vi "picktime.vi"(7 "first":i32 caption="第一", 8 "wdnames":string[](array[string])=["日", "一", "二", "三", "四", "五", "六"] caption="星期名称", 9 "fmtstr":string="%<%X\n%x>T" caption="格式字符串", 10 "secin":timestamp caption="秒输入", 11 "mnames":string[](array[string])=["一月", "二月", "三月", "四月", "五月", "六月", "七月", "八月", "九月", "十月", "十一月", "十二月"] caption="月份名称") -> (1 "ok":bool caption="确定", 2 "secout":timestamp caption="秒输出" format="%<%Z>T")   [LabVIEW 2016]
uses:
  <vilib>/Utility/miscctls.llb/LVPointTypeDef.ctl
panel:
  in  "help":bool caption="取消"
  out "DaylightSavingState":string caption="夏令时状态"
  out "date time rec":T1 caption="日期时间记录"
  in  "Time Display":timestamp caption="时间显示" format="%<%X>T"
  in  "now":bool caption="现在"
  in  "cancel":bool caption="取消"
  in  "ok":bool caption="确定"
  in  "Year":i32=1905 caption="年" min=1600 max=3000
  in  "Month":i32(ring) caption="月" items=["一月", "二月", "三月", "四月", "五月", "六月", "七月", "八月", "九月", "十月", "十一月", "十二月"]
  in  "Date":i32(listbox) caption="日期"
  # "（0表示星期天，1表示星期一，等）"
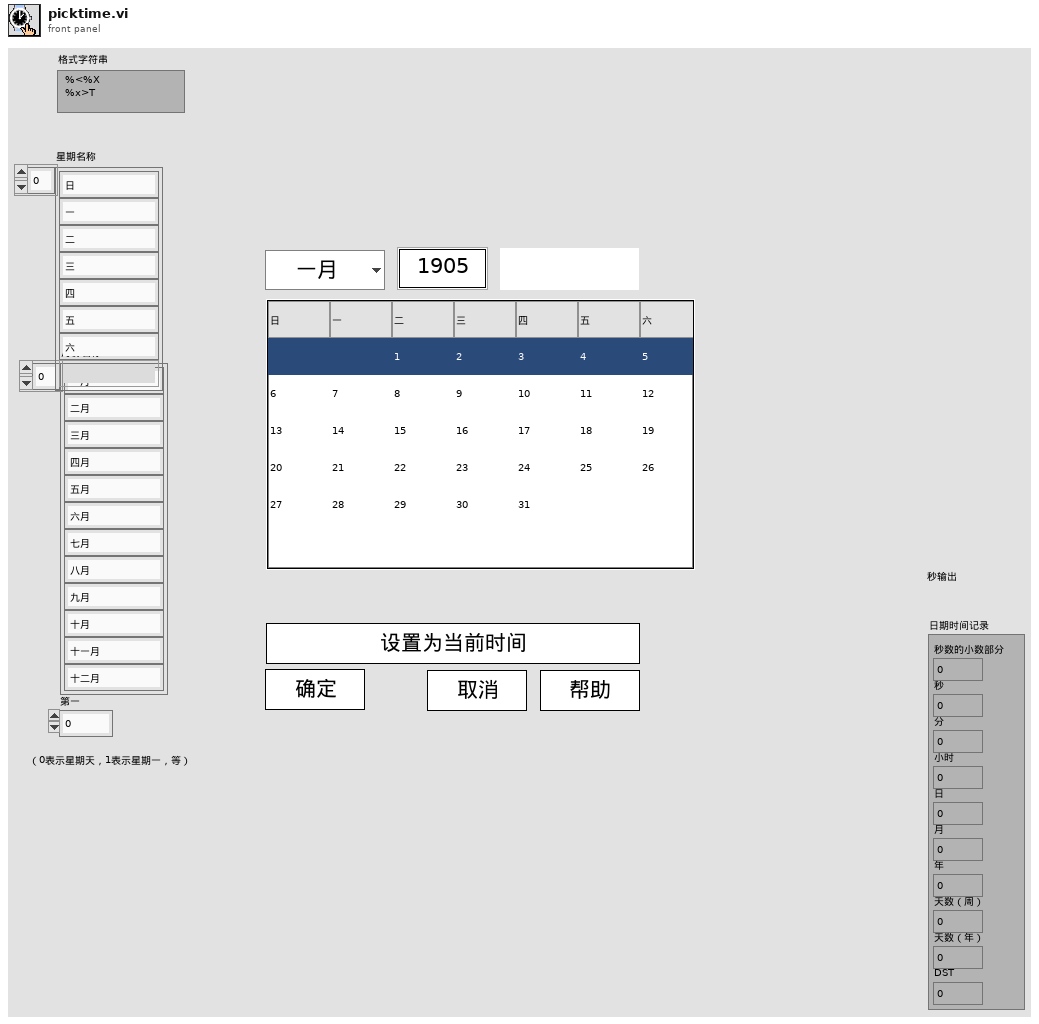
[diagram p1: front panel]
types:
  T1 = cluster{"fractional second":dbl, "second":i32, "minute":i32, "hour":i32, "day of month":i32, "month":i32, "year":i32, "day of week":i32, "day of year":i32, "DST":i32}
  T2 = typedef "LVPointTypeDef.ctl" = cluster{"Horizontal":i16, "Vertical":i16}
  T3 = typedef "LVDateTimeRec.ctl" = cluster{"fractional second":dbl, "second":i32, "minute":i32, "hour":i32, "day of month":i32, "month":i32, "year":i32, "day of week":i32, "day of year":i32, "DST":i32}
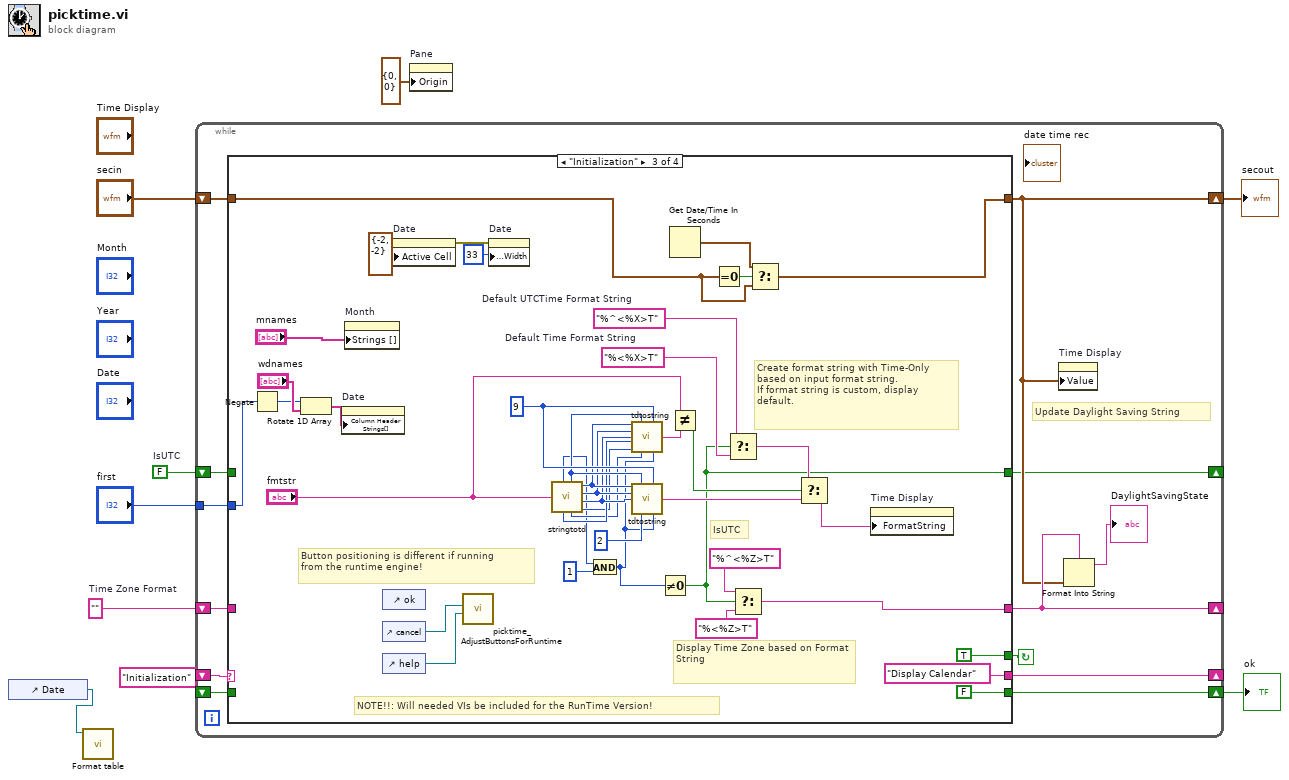
[diagram p0: block diagram]
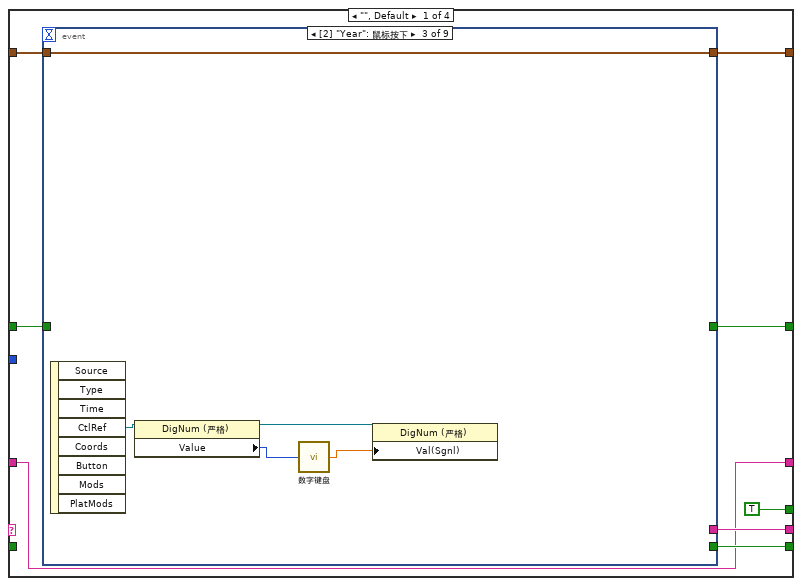
[diagram p2: hidden frame]
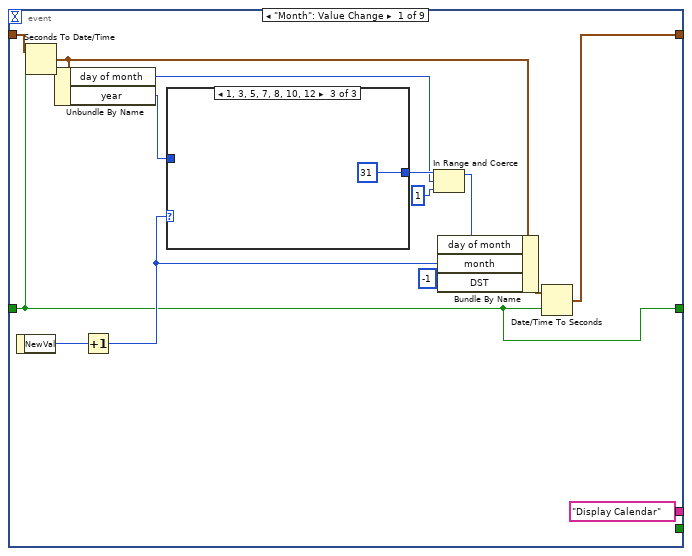
[diagram p3: hidden frame]
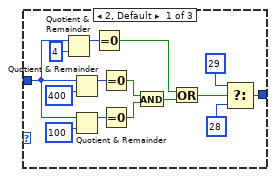
[diagram p4: hidden frame]
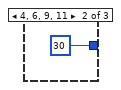
[diagram p5: hidden frame]
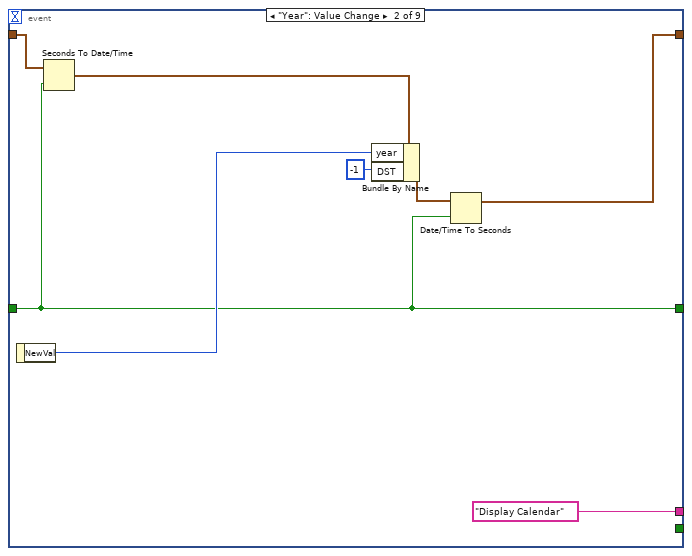
[diagram p6: hidden frame]
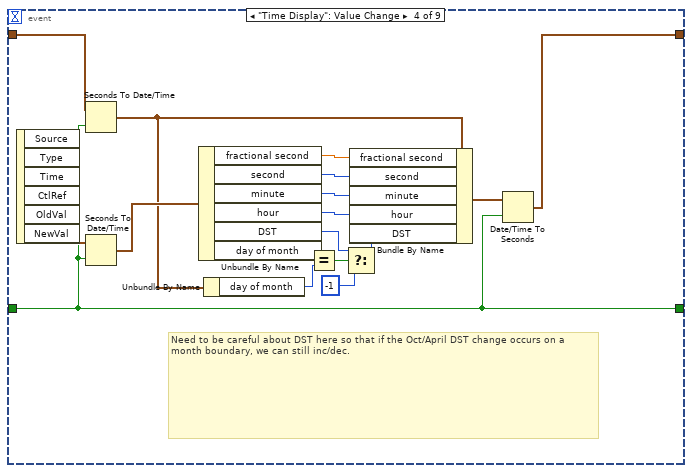
[diagram p7: hidden frame]
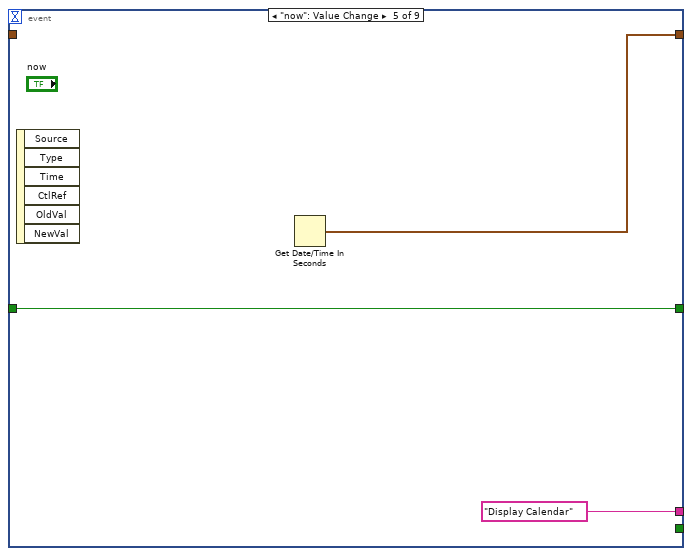
[diagram p8: hidden frame]
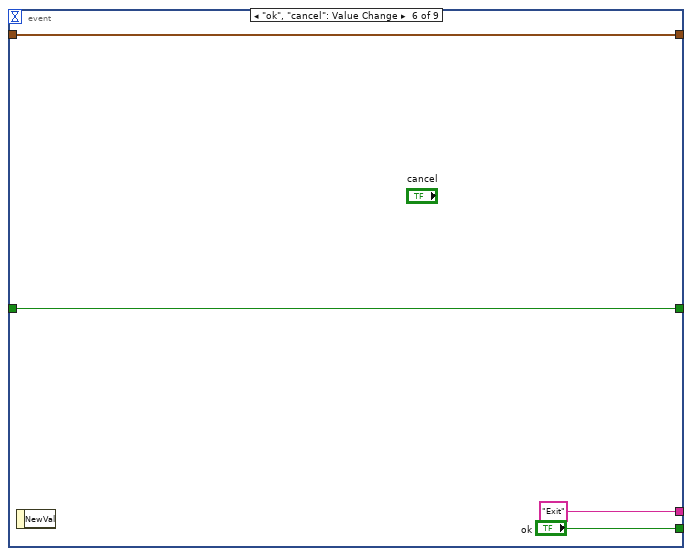
[diagram p9: hidden frame]
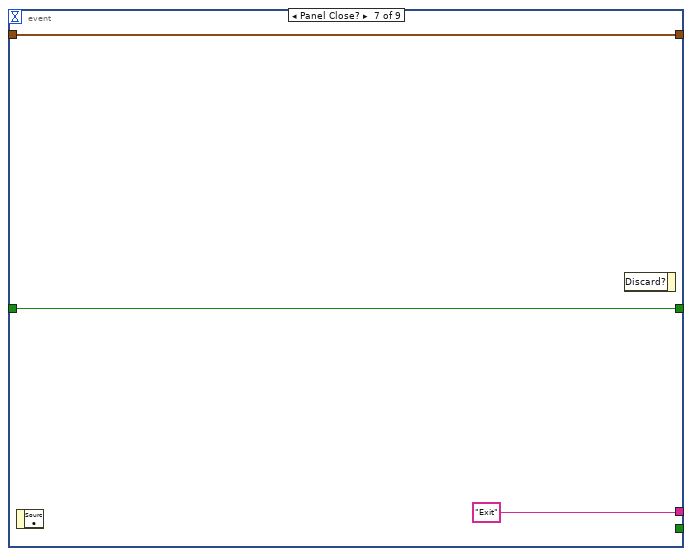
[diagram p10: hidden frame]
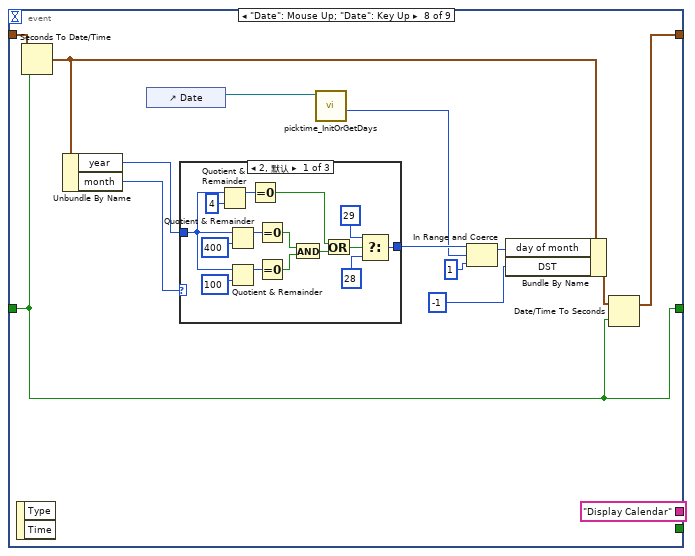
[diagram p11: hidden frame]
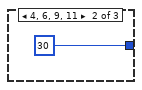
[diagram p12: hidden frame]
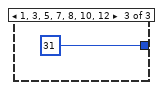
[diagram p13: hidden frame]
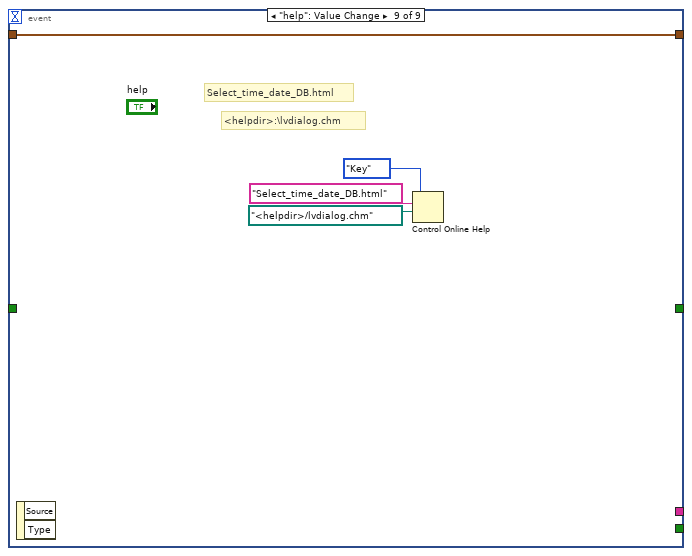
[diagram p14: hidden frame]
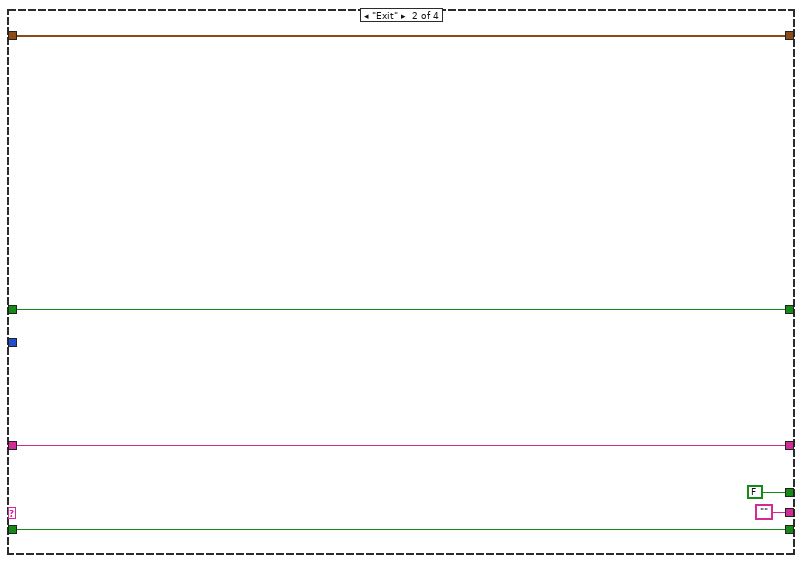
[diagram p15: hidden frame]
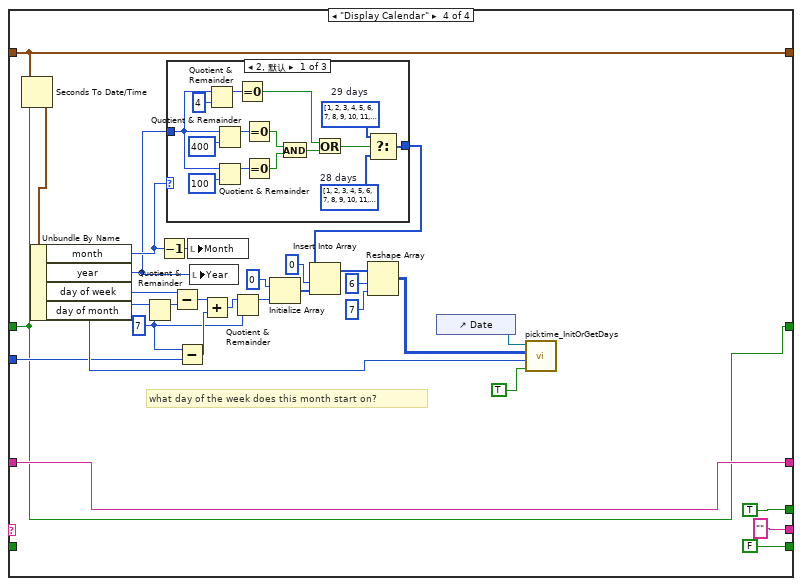
[diagram p16: hidden frame]
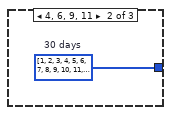
[diagram p17: hidden frame]
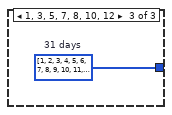
[diagram p18: hidden frame]
diagram:
  w3 = FALSE  # IsUTC
  w5 = ""  # Time Zone Format
  n1 = control-ref of="Date"() -> (w2:refnum<vi>)
  n2 = call "Format table.vi"("Table输入"=w2) -> ()  [unwired: 11 in]
  n3 = while {
    shift-right: [w21] -> _
    shift-left: "Initialization" -> [w22]
    shift-right: [w13] -> w6
    shift-left: "secin" -> [w20]
    shift-right: [w18] -> w8
    shift-left: _ -> [w17]
    shift-right: [w14] -> _
    shift-left: w5 -> [w16]
    tunnel: "first" -> [w12]
    shift-right: [w10] -> _
    shift-left: w3 -> [w11]
    stop <- w19 continue-if-true
    # "Update Daylight Saving String"
    n4 = case shown="\"Initialization\"" w22 {
      tunnel: [w27 "" "Display Calendar" ""] -> w21
      tunnel: [TRUE FALSE TRUE TRUE] -> w19
      tunnel: w20 -> [w28 w139 w174 w194]
      tunnel: [w29 w139 w173 w194] -> w13
      tunnel: [w26 w140 FALSE ("ok") FALSE ("ok")] -> w18
      tunnel: w17 -> [_ w140 _ _]
      tunnel: [w25 w138 w153 w193] -> w14
      tunnel: w16 -> [w25 w138 _ w193]
      tunnel: w12 -> [_ _ w149 w189]
      tunnel: w11 -> [w24 w137 _ w186]
      tunnel: [w23 w137 w147 w186] -> w10
      frame "", Default {
        n5 = event shown="[2] \"Year\": 鼠标按下" {
          selector: _ -> [_ _ _ _ _ _ _ _ _]
          dyn-events: _ -> [_ _ _ _ _ _ _ _ _]
          timeout: _ -> [_ _ _ _ _ _ _ _ _]
          tunnel: w28 -> [w34 w65 w74 w90 _ w96 w100 w107 w136]
          tunnel: [w33 w63 w74 w88 w93 w96 w100 w105 w136] -> w29
          tunnel: ["Display Calendar" "Display Calendar" _ _ "Display Calendar" "Exit" "Exit" "Display Calendar" _] -> w27
          tunnel: [_ _ _ _ _ "ok" _ _ _] -> w26
          tunnel: w24 -> [w31 w62 _ w75 w92 w95 w99 w104 _]
          tunnel: [w31 w62 _ w75 w92 w95 w99 w104 _] -> w23
          event "Month": Value Change {
            n6 = event-data() -> ("NewVal"=w44:i32)  [unwired: 1 out]
            n7 = Seconds To Date/Time(time stamp (now)=w34, to UTC (F)=w31) -> (date time rec=w32:T3)
            n8 = Unbundle By Name(w32) -> ("day of month"=w38:i32, "year"=w39:i32)
            n9 = Increment(x=w44) -> (x+1=w42:i32)
            n10 = case shown="1, 3, 5, 7, 8, 10, 12" w42 {
              tunnel: [w57 30 31] -> w41
              tunnel: w39 -> [w52 _ _]
              frame 2, Default {
                n11 = Quotient & Remainder(x=w52, y=4) -> (x-y*floor(x/y)=w56:i32)  [unwired: 1 out]
                n12 = Quotient & Remainder(x=w52, y=400) -> (x-y*floor(x/y)=w51:i32)  [unwired: 1 out]
                n13 = Quotient & Remainder(x=w52, y=100) -> (x-y*floor(x/y)=w50:i32)  [unwired: 1 out]
                n14 = Equal To 0?(x=w56) -> (x = 0?=w55:bool)
                n15 = Equal To 0?(x=w51) -> (x = 0?=w48:bool)
                n16 = Equal To 0?(x=w50) -> (x = 0?=w49:bool)
                n17 = And(x=w48, y=w49) -> (x .and. y?=w47:bool)
                n18 = Or(x=w55, y=w47) -> (x .or. y?=w54:bool)
                n19 = Select(t=29, s=w54, f=28) -> (s? t:f=w57:i32)
              }
              frame 4, 6, 9, 11 {
              }
              frame 1, 3, 5, 7, 8, 10, 12 {
              }
            }
            n20 = In Range and Coerce(upper limit=w41, x=w38, lower limit=1) -> (coerced(x)=w37:i32)  [unwired: 1 out]
            n21 = Bundle By Name(cluster=w32, "day of month"=w37, "month"=w42, "DST"=-1) -> (w36:T3)
            n22 = Date/Time To Seconds(1:w31, 2:w36) -> (0:w33:timestamp)
          }
          event "Year": Value Change {
            n23 = event-data() -> ("NewVal"=w69:i32)  [unwired: 1 out]
            n24 = Seconds To Date/Time(time stamp (now)=w65, to UTC (F)=w62) -> (date time rec=w64:T3)
            n25 = Bundle By Name(cluster=w64, "year"=w69, "DST"=-1) -> (w67:T3)
            n26 = Date/Time To Seconds(1:w62, 2:w67) -> (0:w63:timestamp)
          }
          event "Year": Mouse Down {
            n27 = event-data() -> ("CtlRef"=w73:refnum<vi>)  [unwired: 8 out]
            n28 = property class="DigNum (严格)"(reference=w73) -> (reference out=w71:refnum<vi>, "Value"=w72:i32)  [unwired: 1 in, 1 out]
            n29 = call "数字键盘.vi"("OldNumber"=w72) -> ("NewNumber"=w70:sgl)
            n30 = property class="DigNum (严格)"(reference=w71, "Val(Sgnl)"=w70) -> ()  [unwired: 1 in, 2 out]
          }
          event "Time Display": Value Change {
            # "Need to be careful about DST here so that if the Oct/April DST change occurs on a month boundary, we can still inc/dec."
            n31 = event-data() -> ("NewVal"=w91:timestamp)  [unwired: 6 out]
            n32 = Seconds To Date/Time(time stamp (now)=w90, to UTC (F)=w75) -> (date time rec=w78:T3)
            n33 = Seconds To Date/Time(time stamp (now)=w91, to UTC (F)=w75) -> (date time rec=w87:T3)
            n34 = Unbundle By Name(w87) -> ("fractional second"=w83:dbl, "second"=w84:i32, "minute"=w85:i32, "hour"=w86:i32, "DST"=w80:i32, "day of month"=w76:i32)
            n35 = Unbundle By Name(w78) -> ("day of month"=w77:i32)
            n36 = Equal?(x=w76, y=w77) -> (x = y?=w82:bool)
            n37 = Select(t=w80, s=w82, f=-1) -> (s? t:f=w79:i32)
            n38 = Bundle By Name(cluster=w78, "fractional second"=w83, "second"=w84, "minute"=w85, "hour"=w86, "DST"=w79) -> (w89:T3)
            n39 = Date/Time To Seconds(1:w75, 2:w89) -> (0:w88:timestamp)
          }
          event "now": Value Change {
            n40 = event-data() -> ()  [unwired: 7 out]
            n41 = Get Date/Time In Seconds() -> (seconds since 1Jan1904=w93:timestamp)
          }
          event "ok", "cancel": Value Change {
            n42 = event-data() -> ()  [unwired: 2 out]
          }
          event Panel Close? {
            n43 = event-data() -> ()  [unwired: 2 out]
            n44 = event-data() -> ()  [unwired: 1 in, 2 out]
          }
          event "Date": Mouse Up; "Date": Key Up {
            n45 = event-data() -> ()  [unwired: 3 out]
            n46 = Seconds To Date/Time(time stamp (now)=w107, to UTC (F)=w104) -> (date time rec=w106:T3)
            n47 = Unbundle By Name(w106) -> ("year"=w113:i32, "month"=w112:i32)
            n48 = control-ref of="Date"() -> (w102:refnum<vi>)
            n49 = case shown="2, 默认" w112 {
              tunnel: [w128 30 31] -> w115
              tunnel: w113 -> [w123 _ _]
              frame 2, Default {
                n50 = Quotient & Remainder(x=w123, y=4) -> (x-y*floor(x/y)=w127:i32)  [unwired: 1 out]
                n51 = Quotient & Remainder(x=w123, y=400) -> (x-y*floor(x/y)=w122:i32)  [unwired: 1 out]
                n52 = Quotient & Remainder(x=w123, y=100) -> (x-y*floor(x/y)=w121:i32)  [unwired: 1 out]
                n53 = Equal To 0?(x=w127) -> (x = 0?=w126:bool)
                n54 = Equal To 0?(x=w122) -> (x = 0?=w119:bool)
                n55 = Equal To 0?(x=w121) -> (x = 0?=w120:bool)
                n56 = And(x=w119, y=w120) -> (x .and. y?=w118:bool)
                n57 = Or(x=w126, y=w118) -> (x .or. y?=w125:bool)
                n58 = Select(t=29, s=w125, f=28) -> (s? t:f=w128:i32)
              }
              frame 4, 6, 9, 11 {
              }
              frame 1, 3, 5, 7, 8, 10, 12 {
              }
            }
            n59 = call <resource>:"picktime_InitOrGetDays.vi"("reference"=w102) -> ("day of month(out)"=w103:i32)  [unwired: 3 in, 7 out]
            n60 = In Range and Coerce(upper limit=w115, x=w103, lower limit=1) -> (coerced(x)=w111:i32)  [unwired: 1 out]
            n61 = Bundle By Name(cluster=w106, "day of month"=w111, "DST"=-1) -> (w109:T3)
            n62 = Date/Time To Seconds(1:w104, 2:w109) -> (0:w105:timestamp)
          }
          event "help": Value Change {
            # "<helpdir>:\\lvdialog.chm"
            # "Select_time_date_DB.html"
            n63 = event-data() -> ()  [unwired: 3 out]
            n64 = Control Online Help(2:path "<helpdir>/lvdialog.chm" ("Path to the help file"), 3:"Select_time_date_DB.html" ("String to search for"), 4:enum16{"Contents", "Key", "Close"}."Key" ("Operation")) -> ()  [unwired: 1 in, 1 out]
          }
        }
      }
      frame "Exit" {
      }
      frame "Initialization" {
        w156 = "%^<%X>T"  # Default UTCTime Format String
        w155 = "%<%X>T"  # Default Time Format String
        w169 = 9 ("Type (9 = Absolute)")
        # "Button positioning is different if running\nfrom the runtime engine!"
        # "IsUTC"
        # "Display Time Zone based on Format String"
        # "NOTE!!: Will needed VIs be included for the RunTime Version!"
        # "Create format string with Time-Only based on input format string.\nIf format string is custom, display default."
        n65 = Negate(x=w149) -> (-x=w148:i32)
        n66 = Rotate 1D Array(1:"wdnames", 2:w148) -> (0:w151:string[])
        n67 = property on="Date" class="MCListbox (严格)"("Column Header Strings[]"=w151) -> ()  [unwired: 2 in, 2 out]
        n68 = property on="Month" class="Ring (严格)"("Strings []"="mnames") -> ()  [unwired: 2 in, 2 out]
        n69 = control-ref of="ok"() -> ()  [unwired: 1 out]
        n70 = control-ref of="cancel"() -> (w144:refnum<vi>)
        n71 = control-ref of="help"() -> (w143:refnum<vi>)
        n72 = property on="Date" class="MCListbox (严格)"("Active Cell"=cluster{i32, i32} {-2, -2}) -> (error out=w181:errorcluster)  [unwired: 2 in, 1 out]
        n73 = call <resource>:"picktime_AdjustButtonsForRuntime.vi"("help button ref"=w143, "cancel button ref"=w144) -> ()  [unwired: 1 in, 9 out]
        n74 = property on="Date" class="MCListbox (严格)"(error in=w181, "Cell Size:Width"=u32 33) -> ()  [unwired: 1 in, 2 out]
        n75 = call <resource>:"stringtotd.vi"("Time & Date Format String"="fmtstr") -> ("UTC"=w145:i16, "MDY"=w164:i16, "Time Format"=w168:i16, "AM/PM"=w167:i16, "included seconds"=w166:i16, "Date Format"=w162:i16, "seconds precision"=w165:i16, "Year Format"=w163:i16)  [unwired: 2 out]
        n76 = And(x=w145, y=i16 1) -> (x .and. y?=w146:i16)
        n77 = call <resource>:"tdtostring.vi"("AM/PM"=w167, "Time Format"=w168, "Type (10 = Absolute)"=w169, "included seconds"=w166, "seconds precision"=w165, "m-d-y sequence"=w164, "year format"=w163, "Date Format"=w162, "UTC"=w146) -> ("Format String"=w160:string)  [unwired: 2 in, 4 out]
        n78 = call <resource>:"tdtostring.vi"("AM/PM"=w167, "Time Format"=w168, "Type (10 = Absolute)"=w169, "included seconds"=w166, "seconds precision"=w165, "Date Format"=i16 2, "UTC"=w146) -> ("Format String"=w158:string)  [unwired: 4 in, 4 out]
        n79 = Not Equal To 0?(x=w146) -> (x != 0?=w147:bool)
        n80 = Get Date/Time In Seconds() -> (seconds since 1Jan1904=w176:timestamp)
        n81 = Not Equal?(x="fmtstr", y=w160) -> (x != y?=w159:bool)
        n82 = Equal To 0?(x=w174) -> (x = 0?=w177:bool)
        n83 = Select(t=w156, s=w147, f=w155) -> (s? t:f=w154:string)
        n84 = Select(t="%^<%Z>T", s=w147, f="%<%Z>T") -> (s? t:f=w153:string)
        n85 = Select(t=w176, s=w177, f=w174) -> (s? t:f=w173:timestamp)
        n86 = Select(t=w154, s=w159, f=w158) -> (s? t:f=w157:string)
        n87 = property on="Time Display" class="AbsTime (严格)"("FormatString"=w157) -> ()  [unwired: 2 in, 2 out]
      }
      frame "Display Calendar" {
        w187 = 7 ("y")
        # "what day of the week does this month start on?"
        n88 = Seconds To Date/Time(time stamp (now)=w194, to UTC (F)=w186) -> (date time rec=w195:T3)
        n89 = Unbundle By Name(w195) -> ("month"=w201:i32, "year"=w200:i32, "day of week"=w211:i32, "day of month"=w192:i32)
        n90 = Quotient & Remainder(x=w192, y=w187) -> (x-y*floor(x/y)=w210:i32)  [unwired: 1 out]
        n91 = Decrement(x=w201) -> (x-1=w202:i32)
        n92 = case shown="2, 默认" w201 {
          tunnel: [w225 w228 w229] -> w196
          tunnel: w200 -> [w218 _ _]
          frame 2, Default {
            w223 = i32[] [1, 2, 3, 4, 5, 6, 7, 8, 9, 10, 11, 12, 13, 14, 15, 16, 17, 18, 19, 20, 21, 22, 23, 24, 25, 26, 27, 28]  # 28 days
            w224 = i32[] [1, 2, 3, 4, 5, 6, 7, 8, 9, 10, 11, 12, 13, 14, 15, 16, 17, 18, 19, 20, 21, 22, 23, 24, 25, 26, 27, 28, 29]  # 29 days
            n93 = Quotient & Remainder(x=w218, y=4) -> (x-y*floor(x/y)=w222:i32)  [unwired: 1 out]
            n94 = Quotient & Remainder(x=w218, y=400) -> (x-y*floor(x/y)=w217:i32)  [unwired: 1 out]
            n95 = Quotient & Remainder(x=w218, y=100) -> (x-y*floor(x/y)=w216:i32)  [unwired: 1 out]
            n96 = Equal To 0?(x=w222) -> (x = 0?=w221:bool)
            n97 = Equal To 0?(x=w217) -> (x = 0?=w214:bool)
            n98 = Equal To 0?(x=w216) -> (x = 0?=w215:bool)
            n99 = And(x=w214, y=w215) -> (x .and. y?=w213:bool)
            n100 = Or(x=w221, y=w213) -> (x .or. y?=w220:bool)
            n101 = Select(t=w224, s=w220, f=w223) -> (s? t:f=w225:i32[])
          }
          frame 4, 6, 9, 11 {
            w228 = i32[] [1, 2, 3, 4, 5, 6, 7, 8, 9, 10, 11, 12, 13, 14, 15, 16, 17, 18, 19, 20, 21, 22, 23, 24, 25, 26, 27, 28, 29, 30]  # 30 days
          }
          frame 1, 3, 5, 7, 8, 10, 12 {
            w229 = i32[] [1, 2, 3, 4, 5, 6, 7, 8, 9, 10, 11, 12, 13, 14, 15, 16, 17, 18, 19, 20, 21, 22, 23, 24, 25, 26, 27, 28, 29, 30, 31]  # 31 days
          }
        }
        n102 = Subtract(x=w211, y=w210) -> (x-y=w191:i32)
        n103 = Subtract(x=w187, y=w189) -> (x-y=w188:i32)
        n104 = local write "Month"(w202) -> ()
        n105 = local write "Year"(w200) -> ()
        n106 = Add(x=w191, y=w188) -> (x+y=w190:i32)
        n107 = Quotient & Remainder(x=w190, y=w187) -> (x-y*floor(x/y)=w199:i32)  [unwired: 1 out]
        n108 = Initialize Array(0, w199) -> (w207:i32[])
        n109 = Insert Into Array(array=w196, index=0, new element=w207) -> (w205:i32[])
        n110 = Reshape Array(w205, 6 ("dimension size"), 7 ("dimension size")) -> (w198:i32[][])
        n111 = control-ref of="Date"() -> (w185:refnum<vi>)
        n112 = call <resource>:"picktime_InitOrGetDays.vi"("Init"=TRUE, "day of month"=w192, "31 days"=w198, "reference"=w185) -> ()  [unwired: 8 out]
      }
    }
    n113 = property on="Time Display" class="AbsTime (严格)"("Value"=w13) -> ()  [unwired: 2 in, 2 out]
    n114 = Format Into String(format string=w14, w13) -> (resulting string=→"DaylightSavingState":string)  [unwired: 2 in, 1 out]
  }
  "ok" <- w8
  "secout" <- w6
  n115 = property on="Pane" class="Pane"("Origin"=T2 {"Horizontal"=0, "Vertical"=0} ("原点")) -> ()  [unwired: 2 in, 2 out]
